vi "Hardware_Power Supplies.vi"(0 "Input VISA":refnum<visa-resource-name>="Power_Supplies", 1 "Power Output ON":bool, 5 "Desired Power":dbl, 7 "Input Resistance":dbl=0.01, 9 "Maximum Power Limit":dbl=10000.0, 11 "Input Error":errorcluster) -> (2 "Output Voltage 1":dbl format="%.4f", 3 "Output Current 1":dbl format="%.4f", 4 "Output VISA":refnum<visa-resource-name>, 6 "Output Power":dbl, 8 "Output Resistance":dbl, 10 "Input Power":dbl, 13 "Output Voltage 2":dbl format="%.4f", 14 "Output Current 2":dbl format="%.4f", 15 "Output Error":errorcluster)   [LabVIEW 2017]
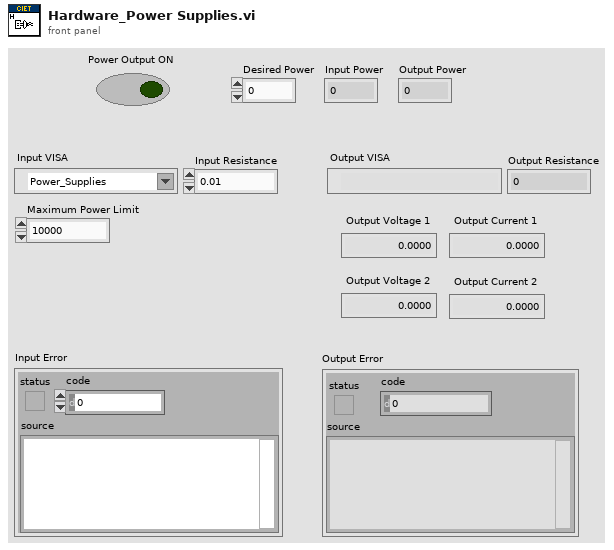
[diagram p1: front panel]
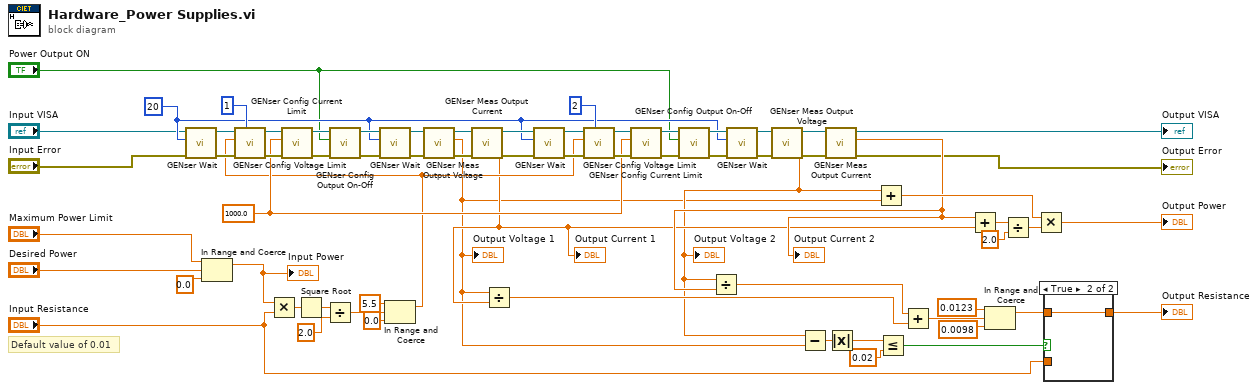
[diagram p0: block diagram]
diagram:
  w31 = u32 20 ("Delay (20 mS)")
  w41 = 1000.0 ("Current Limit")
  # "Default value of 0.01"
  n1 = call "GENser Wait.vi"("error"="Input Error", "Delay (20 mS)"=w31, "VISA"="Input VISA") -> ("error out"=w55:errorcluster, "VISA out"=w54:refnum<visa-resource-name>)  [unwired: 7 in]
  n2 = In Range and Coerce(upper limit="Maximum Power Limit", x="Desired Power", lower limit=0.0) -> (coerced(x)=w25:dbl)  [unwired: 1 out]
  "Input Power" <- w25
  n3 = Multiply(x=w25, y="Input Resistance") -> (x*y=w39:dbl)
  n4 = Square Root(x=w39) -> (sqrt(x)=w38:dbl)
  n5 = Divide(x=w38, y=2.0) -> (x/y=w34:dbl)
  n6 = In Range and Coerce(upper limit=5.5, x=w34, lower limit=0.0) -> (coerced(x)=w26:dbl)  [unwired: 1 out]
  n7 = call "GENser Config Voltage Limit.vi"("GEN Addr"=i16 1, "error"=w55, "Volt Limit"=w26, "VISA"=w54) -> ("error out"=w67:errorcluster, "VISA out"=w53:refnum<visa-resource-name>)  [unwired: 6 in]
  n8 = call "GENser Config Current Limit.vi"("error"=w67, "Current Limit"=w41, "VISA"=w53) -> ("error out"=w64:errorcluster, "VISA out"=w52:refnum<visa-resource-name>)  [unwired: 7 in]
  n9 = call "GENser Config Output On-Off.vi"("error"=w64, "Output ON"="Power Output ON", "VISA"=w52) -> ("error out"=w62:errorcluster, "VISA out"=w51:refnum<visa-resource-name>)  [unwired: 7 in]
  n10 = call "GENser Wait.vi"("error"=w62, "Delay (20 mS)"=w31, "VISA"=w51) -> ("error out"=w61:errorcluster, "VISA out"=w50:refnum<visa-resource-name>)  [unwired: 7 in]
  n11 = call "GENser Meas Output Voltage.vi"("error"=w61, "VISA"=w50) -> ("error out"=w63:errorcluster, "Output Voltage"=w11:dbl, "VISA out"=w49:refnum<visa-resource-name>)  [unwired: 7 in]
  "Output Voltage 1" <- w11
  n12 = call "GENser Meas Output Current.vi"("error"=w63, "VISA"=w49) -> ("error out"=w59:errorcluster, "Output Current"=w15:dbl, "VISA out"=w48:refnum<visa-resource-name>)  [unwired: 7 in]
  "Output Current 1" <- w15
  n13 = Divide(x=w11, y=w15) -> (x/y=w13:dbl)
  n14 = call "GENser Wait.vi"("error"=w59, "Delay (20 mS)"=w31, "VISA"=w48) -> ("error out"=w58:errorcluster, "VISA out"=w47:refnum<visa-resource-name>)  [unwired: 7 in]
  n15 = call "GENser Config Voltage Limit.vi"("GEN Addr"=i16 2, "error"=w58, "Volt Limit"=w26, "VISA"=w47) -> ("error out"=w60:errorcluster, "VISA out"=w46:refnum<visa-resource-name>)  [unwired: 6 in]
  n16 = call "GENser Config Current Limit.vi"("error"=w60, "Current Limit"=w41, "VISA"=w46) -> ("error out"=w57:errorcluster, "VISA out"=w45:refnum<visa-resource-name>)  [unwired: 7 in]
  n17 = call "GENser Config Output On-Off.vi"("error"=w57, "Output ON"="Power Output ON", "VISA"=w45) -> ("error out"=w66:errorcluster, "VISA out"=w44:refnum<visa-resource-name>)  [unwired: 7 in]
  n18 = call "GENser Wait.vi"("error"=w66, "Delay (20 mS)"=w31, "VISA"=w44) -> ("error out"=w56:errorcluster, "VISA out"=w43:refnum<visa-resource-name>)  [unwired: 7 in]
  n19 = call "GENser Meas Output Voltage.vi"("error"=w56, "VISA"=w43) -> ("error out"=w65:errorcluster, "Output Voltage"=w12:dbl, "VISA out"=w42:refnum<visa-resource-name>)  [unwired: 7 in]
  "Output Voltage 2" <- w12
  n20 = Subtract(x=w12, y=w11) -> (x-y=w21:dbl)
  n21 = call "GENser Meas Output Current.vi"("error"=w65, "VISA"=w42) -> ("error out"=→"Output Error":errorcluster, "Output Current"=w16:dbl, "VISA out"=→"Output VISA":refnum<visa-resource-name>)  [unwired: 7 in]
  "Output Current 2" <- w16
  n22 = Divide(x=w12, y=w16) -> (x/y=w14:dbl)
  n23 = Absolute Value(x=w21) -> (abs(x)=w20:dbl)
  n24 = Add(x=w12, y=w11) -> (x+y=w27:dbl)
  n25 = Less Or Equal?(x=w20, y=0.02) -> (x <= y?=w18:bool)
  n26 = Add(x=w14, y=w13) -> (x+y=w22:dbl)
  n27 = Add(x=w16, y=w15) -> (x+y=w30:dbl)
  n28 = In Range and Coerce(upper limit=0.0123, x=w22, lower limit=0.0098) -> (coerced(x)=w17:dbl)  [unwired: 1 out]
  n29 = Divide(x=w30, y=2.0) -> (x/y=w28:dbl)
  n30 = Multiply(x=w27, y=w28) -> (x*y=→"Output Power":dbl)
  n31 = case shown="True" w18 {
    tunnel: w17 -> [_ w69]
    tunnel: [w68 w69] -> w8
    tunnel: "Input Resistance" -> [w68 _]
    frame False {
    }
    frame True {
    }
  }
  "Output Resistance" <- w8
